vi "write_params.vi"(8 "error in (no error)":errorcluster, 10 "params":T1={"estimators"=[], "voting"="hard", "weights"={"weights_type"="None", "weights_list"=[]}, "n_jobs"=1.0, "flatten_transform"=TRUE, "verbose"=FALSE}, 11 "VotingClassifier in":refnum<class "VotingClassifier.lvclass">) -> (0 "error out":errorcluster, 3 "VotingClassifier out":refnum<class "VotingClassifier.lvclass">)   [LabVIEW 2020, in "VotingClassifier.lvclass"]
uses:
  VotingClassifier.lvclass
  Controls/voting_classifier_params.ctl
  VotingClassifier.lvclass/VotingClassifier.ctl
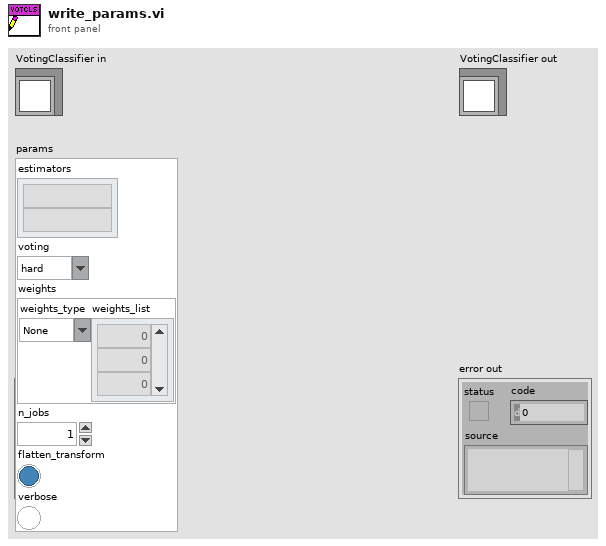
[diagram p1: front panel]
types:
  T1 = typedef "voting_classifier_params.ctl" = cluster{"estimators":string[], "voting":string, "weights":cluster{"weights_type":string, "weights_list":dbl[]}, "n_jobs":dbl, "flatten_transform":bool, "verbose":bool}
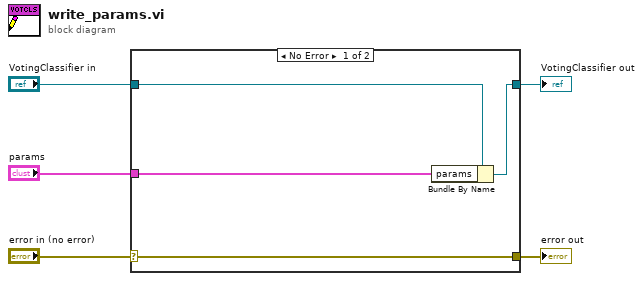
[diagram p0: block diagram]
diagram:
  n1 = case shown="No Error" "error in (no error)" {
    selector: "error in (no error)" -> [w9 w10]
    tunnel: [w9 w10] -> w4
    tunnel: [w7 w11] -> w2
    tunnel: "VotingClassifier in" -> [w8 w11]
    tunnel: "params" -> [w6 _]
    frame No Error {
      n2 = Bundle By Name(cluster=w8, "params"=w6) -> (w7:refnum<class "VotingClassifier.lvclass">)
    }
    frame Error {
    }
  }
  "error out" <- w4
  "VotingClassifier out" <- w2
